vi "MeasResSummToInsertZ JH.vi"(4 "floating-point type conversion":string[][](table)=[["extended", "5", "12"], ["double", "5", "9"], ["single", "5", "5"]], 6 "error in":T2, 7 "create dynamic SQL":bool, 8 "temperature":T1 {"temperatureC" format="%.2f"; "pulseVoltage" format="%.3f"; "scanRange" format="%.3f"; "pulseRepetRate" format="%.3f"; "txpgWaveformStyle" format="%.3f"; "roomTempC" format="%.2f"; "txFrequencyHz" format="%.3f"; "numTxCycles" format="%.1f"; "probeId" format="%#.0f"}, 9 "connection reference":refnum<k7>) -> (0 "error out":T2, 1 "insert sql statement":string, 3 "connection reference":refnum<k7>)   [LabVIEW 2016]
doc: "This VI will dynamically create an INSERT SQL statement for meas_res_summary."
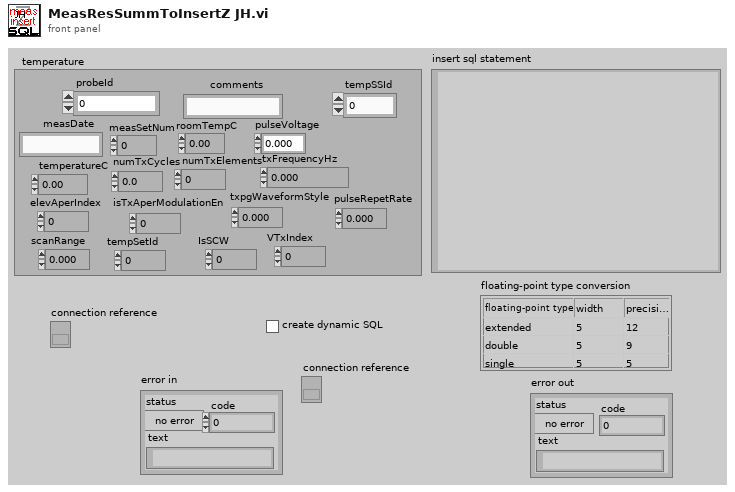
[diagram p1: front panel]
types:
  T1 = cluster{"probeId":dbl, "comments":string, "tempSSId":i16, "measDate":string, "measSetNum":i16, "roomTempC":sgl, "pulseVoltage":dbl, "temperatureC":ext, "numTxCycles":dbl, "numTxElements":i16, "txFrequencyHz":dbl, "elevAperIndex":i16, "isTxAperModulationEn":i16, "txpgWaveformStyle":sgl, "pulseRepetRate":sgl, "scanRange":sgl, "tempSetId":i16, "IsSCW":i16, "VTxIndex":i16}
  T2 = cluster{"status":bool, "code":i32, "text":string}
  T3 = cluster{"name":string, "type  ":u16, "value":string}[]
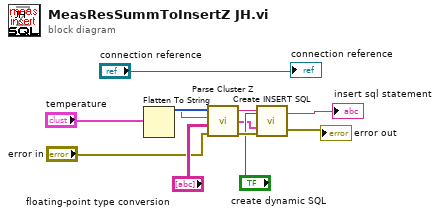
[diagram p0: block diagram]
diagram:
  n1 = Flatten To String(anything="temperature") -> (data string=w10:string, type string=w11:i16[])  [unwired: 3 in, 1 out]
  n2 = call "Parse Cluster Z.vi"("error in"="error in", "floating-point type conversion"="floating-point type conversion", "cluster data"=w10, "cluster definition"=w11) -> ("error out"=w7:T2, "cluster controls"=w4:T3, "cluster name"=w8:string)
  n3 = call <vilib>:"Create INSERT SQL.vi"("error in"=w7, "column info"=w4, "create dynamic SQL"="create dynamic SQL", "table name"=w8) -> ("error out"=→"error out":errorcluster, "SQL insert statement"=→"insert sql statement":string)
  "connection reference" <- "connection reference"
